vi "init.vi"(8 "error in (no error)":errorcluster, 11 "car in":refnum<class "car.lvclass">) -> (0 "error out":errorcluster, 3 "car out":refnum<class "car.lvclass">)   [LabVIEW 2011, in "car.lvclass"]
uses:
  car.lvclass
  genericVehicle/vehicleGeneric.lvclass
  car.lvclass/car.ctl
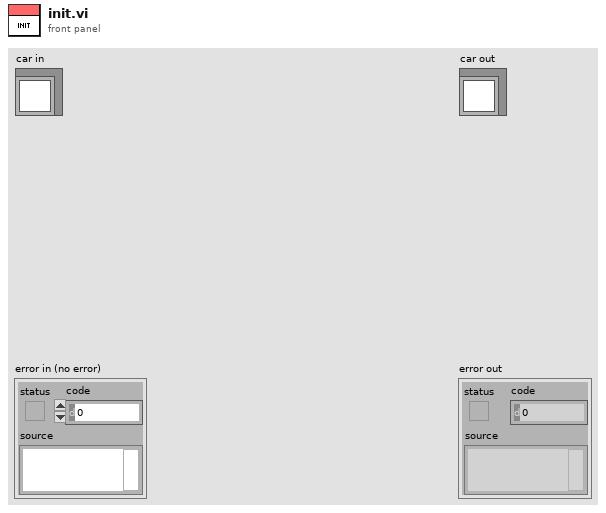
[diagram p1: front panel]
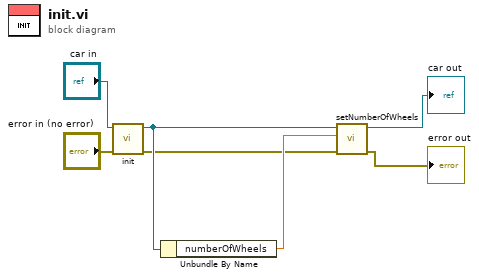
[diagram p0: block diagram]
diagram:
  n1 = call-parent "init.vi"("error in (no error)"="error in (no error)", "vehicleGeneric in"="car in") -> ("error out"=w2:errorcluster, "vehicleGeneric out"=w5:refnum<class "car.lvclass">)  [unwired: 8 in]
  n2 = Unbundle By Name(w5) -> ("numberOfWheels"=w3:dbl)
  n3 = call-dynamic "setNumberOfWheels.vi"("error in (no error)"=w2, "numberOfWheels"=w3, "vehicleGeneric in"=w5) -> ("error out"=→"error out":errorcluster, "vehicleGeneric out"=→"car out":refnum<class "car.lvclass">)  [unwired: 7 in]
